vi "Self-Test.vi"(8 "Error in (no error)":errorcluster, 11 "VISA resource":refnum<visa-resource-name>) -> (0 "Error out":errorcluster, 2 "Self-test response":string, 3 "Dup VISA resource":refnum<visa-resource-name>)   [LabVIEW 2010]
doc: "Copyright (c) 2012 Metrolab Technology SA, Plan-les-Ouates, Geneva, Switzerland\nRun instrument self-test.\nNote: the THM1176 does not support self-test."
panel:
  # "Self-Test"
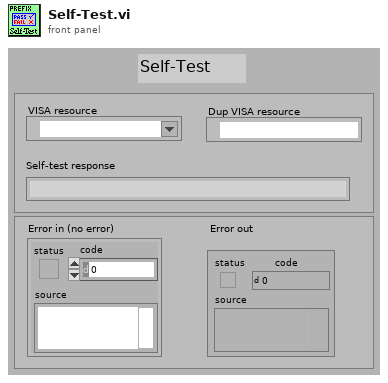
[diagram p1: front panel]
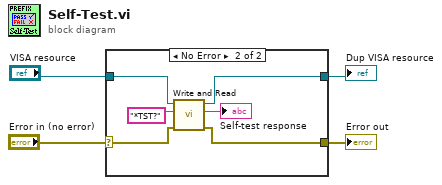
[diagram p0: block diagram]
diagram:
  n1 = case shown="No Error" "Error in (no error)" {
    selector: "Error in (no error)" -> [w5 w11]
    tunnel: [w5 w8] -> w3
    tunnel: [w6 w9] -> w1
    tunnel: "VISA resource" -> [w6 w10]
    frame Error {
    }
    frame No Error {
      n2 = call "Write and Read.vi"("Error in (no error)"=w11, "Command"="*TST?", "VISA resource"=w10) -> ("Error out"=w8:errorcluster, "Response"=→"Self-test response":string, "Dup VISA resource"=w9:refnum<visa-resource-name>)  [unwired: 4 in, 2 out]
    }
  }
  "Error out" <- w3
  "Dup VISA resource" <- w1
